vi "ReadDataMK4.vi"(9 "millisecondIN":u32, 11 "input cluster":T1) -> (1 "millisecondOUT":u32, 2 "STATEUART":T3, 3 "Cluster":T2)   [LabVIEW 2017]
uses:
  mWorkToolkit/libSerial/STATEUART.ctl
  mWorkToolkit/libSerial/stateSerialUltra.ctl
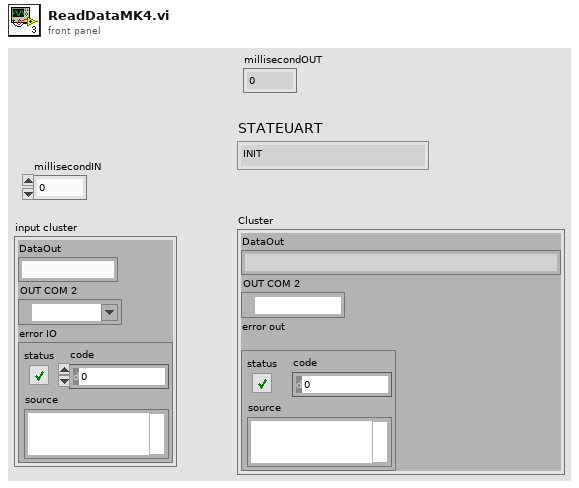
[diagram p1: front panel]
types:
  T1 = cluster{"DataOut":string, "OUT COM 2":refnum<visa-resource-name>, "error IO":errorcluster}
  T2 = cluster{"DataOut":string, "OUT COM 2":refnum<visa-resource-name>, "error out\n":errorcluster}
  T3 = typedef "STATEUART.ctl" = enum16{"INIT", "WRITE", "READ", "CHECKDATA", "IDLE", "STOP"}
  T4 = typedef "stateSerialUltra.ctl" = enum16{"findCOM", "Init", "CheckConnect", "Read", "Write", "exit"}
  T5 = cluster{string, "OUT COM 2":refnum<visa-resource-name>, "error out":errorcluster}
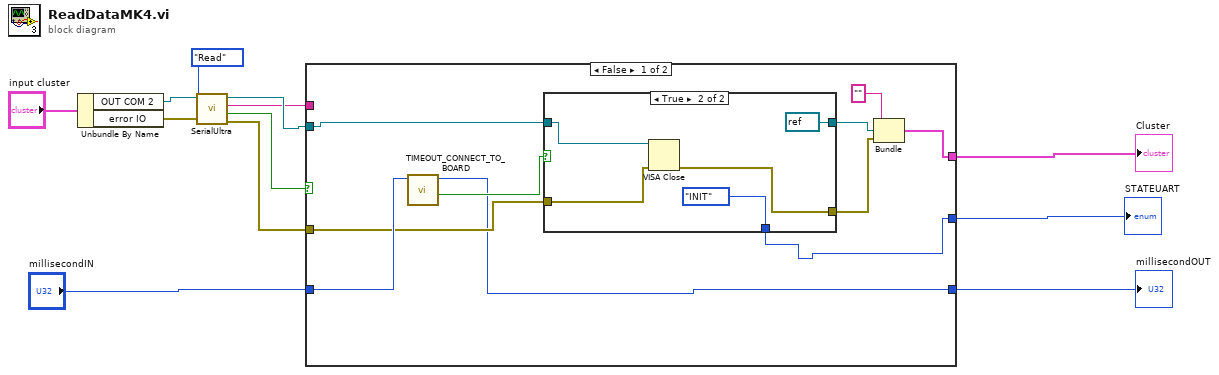
[diagram p0: block diagram]
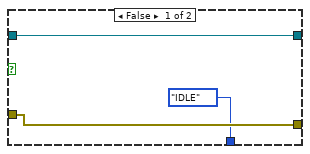
[diagram p2: hidden frame]
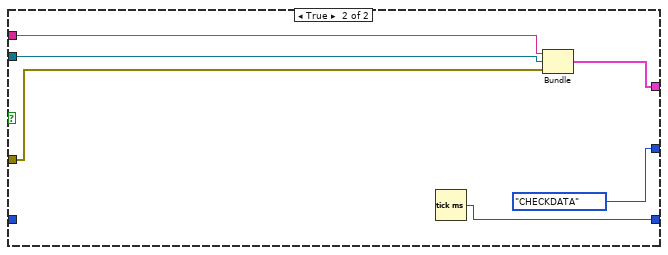
[diagram p3: hidden frame]
diagram:
  n1 = Unbundle By Name("input cluster") -> ("OUT COM 2"=w9:refnum<visa-resource-name>, "error IO"=w8:errorcluster)
  n2 = call "SerialUltra.vi"("error in"=w8, "State"=stateSerialUltra."Read", "IN COM"=w9) -> ("error out"=w10:errorcluster, "IsData"=w11:bool, "DataOut"=w6:string, "OUT COM 2"=w7:refnum<visa-resource-name>)  [unwired: 4 in, 1 out]
  n3 = case shown="False" w11 {
    tunnel: w10 -> [w20 w33]
    tunnel: "millisecondIN" -> [w22 _]
    tunnel: [w19 w36] -> w4
    tunnel: [w18 STATEUART."CHECKDATA"] -> w5
    tunnel: [w16 w32] -> w3
    tunnel: w7 -> [w17 w34]
    tunnel: w6 -> [_ w31]
    frame False {
      n4 = call "TIMEOUT_CONNECT_TO_BOARD.vi"("TIMEBEGIN"=w22) -> ("STATUS"=w21:bool, "TIMEOUT"=w19:u32)  [unwired: 9 in]
      n5 = case shown="True" w21 {
        tunnel: w17 -> [w23 w30]
        tunnel: w20 -> [w25 w29]
        tunnel: [w25 w28] -> w14
        tunnel: [STATEUART."IDLE" STATEUART."INIT"] -> w18
        tunnel: [w23 refnum<visa-resource-name> refnum ("OUT COM 2")] -> w15
        frame False {
        }
        frame True {
          n6 = VISA Close(VISA resource name=w30, error in (no error)=w29) -> (error out=w28:errorcluster)
        }
      }
      n7 = Bundle("", "OUT COM 2"=w15, "error out"=w14) -> (w16:T5)  [unwired: 1 in]
    }
    frame True {
      n8 = Tick Count (ms)() -> (millisecond timer value=w36:u32)
      n9 = Bundle("DataOut"=w31, "OUT COM 2"=w34, "error out"=w33) -> (w32:T2)  [unwired: 1 in]
    }
  }
  "STATEUART" <- w5
  "millisecondOUT" <- w4
  "Cluster" <- w3
